vi "Exemple 1.vi"() -> ()   [LabVIEW 2018]
panel:
  out "C":dbl
  in  "B":dbl
  in  "A":dbl
  # "Exemple 1: calcul c=2(a+b)(a-3b)"
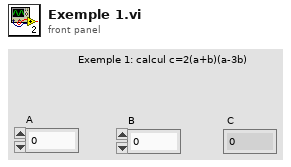
[diagram p1: front panel]
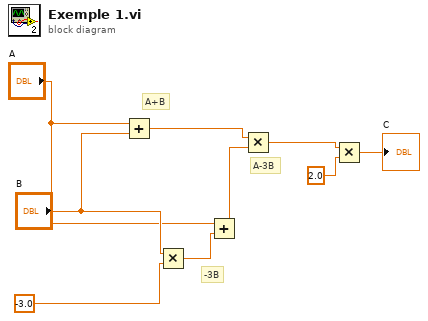
[diagram p0: block diagram]
diagram:
  # "A-3B"
  # "-3B"
  # "A+B"
  n1 = Add(x="A", y="B") -> (x+y=w5:dbl)
  n2 = Multiply(x="B", y=-3.0) -> (x*y=w6:dbl)
  n3 = Add(x="A", y=w6) -> (x+y=w4:dbl)
  n4 = Multiply(x=w5, y=w4) -> (x*y=w3:dbl)
  n5 = Multiply(x=w3, y=2.0) -> (x*y=→"C":dbl)
